vi "InitializeMission.vi"(4 "Tolerance (m)":dbl, 5 "Done":bool, 6 "Timeout (s)":dbl=-1.0, 7 "Duration (s)":dbl=-1.0, 8 "Error In":errorcluster, 9 "Points of Interest":T1[](array[typedef]) {"North" format="%#_10f"; "East" format="%#_8f"}, 10 "Mission Type":T2, 11 "StationKeeping in":refnum<class "StationKeeping.lvclass">) -> (0 "Error Out":errorcluster, 3 "StationKeeping out":refnum<class "StationKeeping.lvclass">)   [LabVIEW 2013, in "StationKeeping.lvclass"]
uses:
  StationKeeping.lvclass
  Data/TypeDefs/MissionTypeControl.ctl
  Data/TypeDefs/UTM Location.ctl
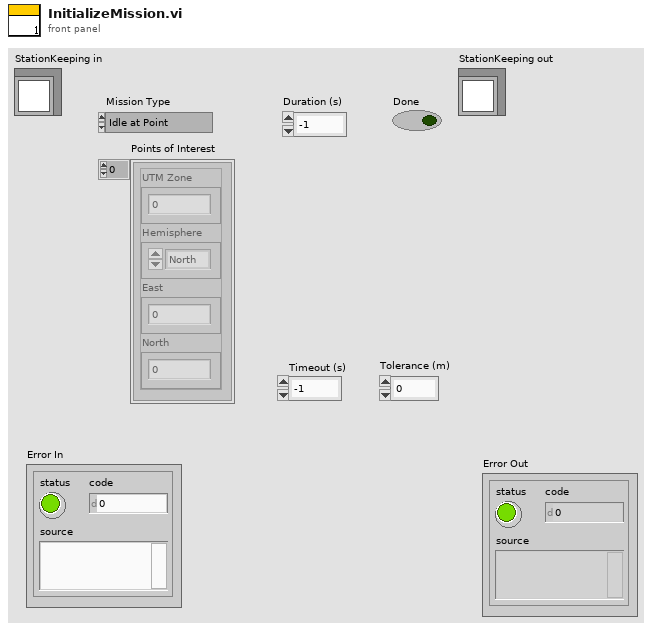
[diagram p1: front panel]
types:
  T1 = typedef "UTM Location.ctl" = cluster{"UTM Zone":dbl, "Hemisphere":enum16{"North", "South"}, "East":dbl, "North":dbl}
  T2 = typedef "MissionTypeControl.ctl" = enum16{"Idle at Point", "Drive to Waypoint", "Round Buoy to Port", "Round Buoy to Starboard", "Pass Between Buoys", "Station Keeping"}
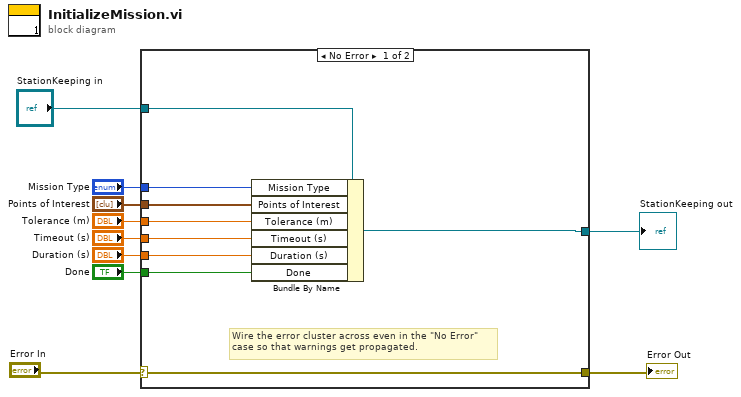
[diagram p0: block diagram]
diagram:
  n1 = case shown="No Error" "Error In" {
    selector: "Error In" -> [w19 w21]
    tunnel: [w19 w21] -> w2
    tunnel: [w11 w20] -> w9
    tunnel: "StationKeeping in" -> [w12 w20]
    tunnel: "Mission Type" -> [w18 _]
    tunnel: "Points of Interest" -> [w17 _]
    tunnel: "Tolerance (m)" -> [w16 _]
    tunnel: "Timeout (s)" -> [w15 _]
    tunnel: "Duration (s)" -> [w14 _]
    tunnel: "Done" -> [w13 _]
    frame No Error {
      # "Wire the error cluster across even in the \"No Error\"\ncase so that warnings get propagated."
      n2 = Bundle By Name(cluster=w12, "Mission Type"=w18, "Points of Interest"=w17, "Tolerance (m)"=w16, "Timeout (s)"=w15, "Duration (s)"=w14, "Done"=w13) -> (w11:refnum<class "StationKeeping.lvclass">)
    }
    frame Error {
    }
  }
  "StationKeeping out" <- w9
  "Error Out" <- w2
